vi "Export Filtered Mappings.vi"(8 "error in (no error)":errorcluster, 9 "Filtered Node":string, 10 "Path":path, 11 "SDF Ref":refnum<k24>) -> (0 "error out":errorcluster)   [LabVIEW 2016, in "System Mapping Tool.lvlib"]
uses:
  System Mapping Tool.lvlib
  NationalInstruments.VeriStand.SystemDefinitionAPI
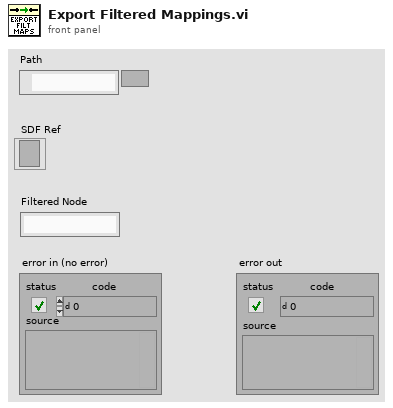
[diagram p1: front panel]
types:
  T1 = enum16{"open", "replace", "create", "open or create", "replace or create", "replace or create with confirmation"}
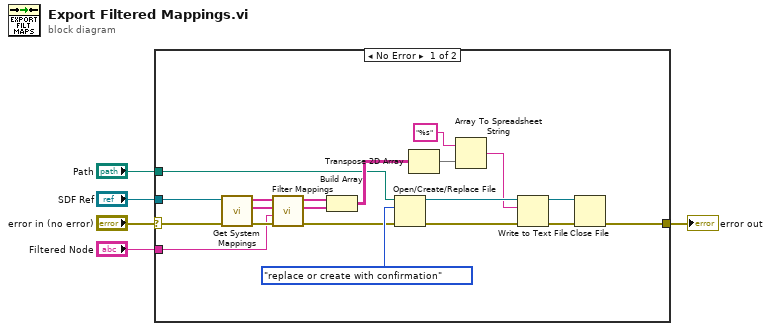
[diagram p0: block diagram]
diagram:
  n1 = case shown="No Error" "error in (no error)" {
    selector: "error in (no error)" -> [w17 w26]
    tunnel: [w14 w26] -> w4
    tunnel: "SDF Ref" -> [w16 _]
    tunnel: "Path" -> [w13 _]
    tunnel: "Filtered Node" -> [w9 _]
    frame No Error {
      n2 = call "Get System Mappings.vi"("error in (no error)"=w17, "SDF Ref"=w16) -> ("error out"=w12:errorcluster, "Destinations"=w10:string[], "Sources"=w11:string[])  [unwired: 7 in]
      n3 = call "Filter Mappings.vi"("error in (no error)"=w12, "Path to Filter"=w9, "Destinations"=w10, "Sources"=w11) -> ("error out"=w8:errorcluster, "Filtered Destinations"=w6:string[], "Filtered Sources"=w7:string[])  [unwired: 5 in]
      n4 = Build Array(w7, w6) -> (w24:string[][])
      n5 = Open/Create/Replace File(file path (use dialog)=w13, error in=w8, operation (0:open)=T1."replace or create with confirmation") -> (refnum out=w22:refnum<file>, error out=w15:errorcluster)  [unwired: 3 in, 1 out]
      n6 = Transpose 2D Array(2D array=w24) -> (transposed array=w18:string[][])
      n7 = Array To Spreadsheet String(array=w18, 3:"%s" ("format string")) -> (spreadsheet string=w21:string)  [unwired: 1 in]
      n8 = Write to Text File(file (use dialog)=w22, text=w21, error in=w15) -> (refnum out=w19:refnum<file>, error out=w20:errorcluster)  [unwired: 1 in, 1 out]
      n9 = Close File(refnum=w19, error in=w20) -> (error out=w14:errorcluster)  [unwired: 1 out]
    }
    frame Error {
    }
  }
  "error out" <- w4
